vi "Points to Line Descriptor.vi"(10 "Y":i16[](array[numeric]), 11 "X":i16[](array[numeric])) -> (3 "Line out":T1)   [LabVIEW 2011]
uses:
  Line Descriptor.ctl
  <vilib>/Analysis/NI_AALPro.lvlib
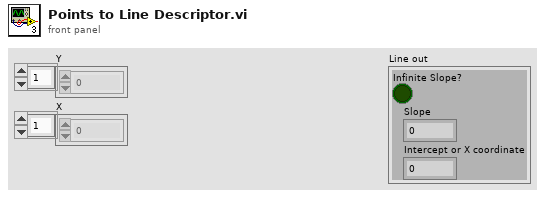
[diagram p1: front panel]
types:
  T1 = cluster{"Infinite Slope?":bool, "Slope":dbl, "Intercept or X coordinate":dbl}
  T2 = typedef "Line Descriptor.ctl" = cluster{"Infinite Slope?":bool, "Slope":dbl, "Intercept or X coordinate":dbl}
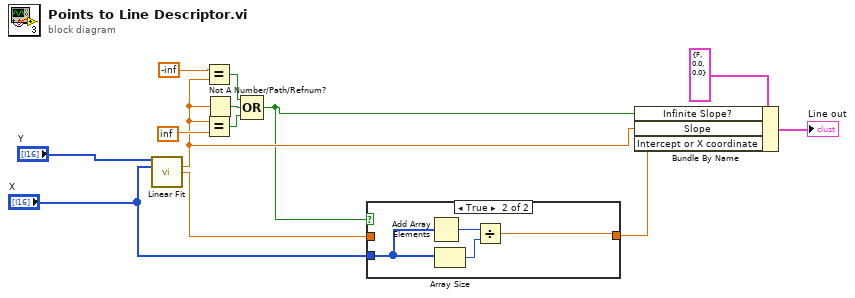
[diagram p0: block diagram]
diagram:
  n1 = call <vilib>:"Linear Fit.vi"("Y"="Y", "X"="X") -> ("slope"=w3:dbl, "intercept"=w12:dbl)  [unwired: 9 in, 3 out]
  n2 = Equal?(x=-inf, y=w3) -> (x = y?=w8:bool)
  n3 = Equal?(x=w3, y=inf) -> (x = y?=w7:bool)
  n4 = Not A Number/Path/Refnum?(number/path/refnum=w3) -> (NaN/Path/Refnum?=w9:bool)
  n5 = Compound Arithmetic op=OR(w8, w9, w7) -> (w2:bool)
  n6 = case shown="True" w2 {
    tunnel: w12 -> [w14 _]
    tunnel: "X" -> [_ w18]
    tunnel: [w14 w15] -> w4
    frame False {
    }
    frame True {
      n7 = Add Array Elements(numeric array=w18) -> (sum=w17:i16)
      n8 = Array Size(array=w18) -> (size(s)=w16:i32)
      n9 = Divide(x=w17, y=w16) -> (x/y=w15:dbl)
    }
  }
  n10 = Bundle By Name(cluster=T2 {"Infinite Slope?"=FALSE, "Slope"=0.0, "Intercept or X coordinate"=0.0} ("Line Descriptor"), "Infinite Slope?"=w2, "Slope"=w3, "Intercept or X coordinate"=w4) -> (→"Line out":T2)
